vi "ziGetVoltage.vi"(4 "DemodVoltage (Vrms)":cdb[](array[numeric]) format="%#_6p", 6 "ZCtrl / Gain (0)":dbl, 8 "error in":errorcluster, 9 "Demodulator (0)":i32, 10 "Mode":enum16{"From Sig Out", "Signal Input", "HF2CA"}(ring), 11 "handle in":T1 {"Handle" format="0x%08x"; "Conn" format="0x%08x"}) -> (0 "error out":errorcluster, 2 "Vz (Vrms)":cdb[](array[numeric]) format="%#_6p", 3 "handle out":T1 {"Handle" format="0x%08x"; "Conn" format="0x%08x"})   [LabVIEW 2009, in "Zurich Instruments LabOne.lvlib"]
doc: "Get the effective voltage from measured demod samples."
uses:
  <instrlib>/Zurich Instruments LabOne/Zurich Instruments LabOne.lvlib
  <instrlib>/Zurich Instruments LabOne/Public/ziTypeHandle.ctl
  <instrlib>/Zurich Instruments LabOne/Public/Utility/Impedance/ziGetVoltageCalcVec.vi
panel:
  in  "Extra Gain (1)":dbl=1.0
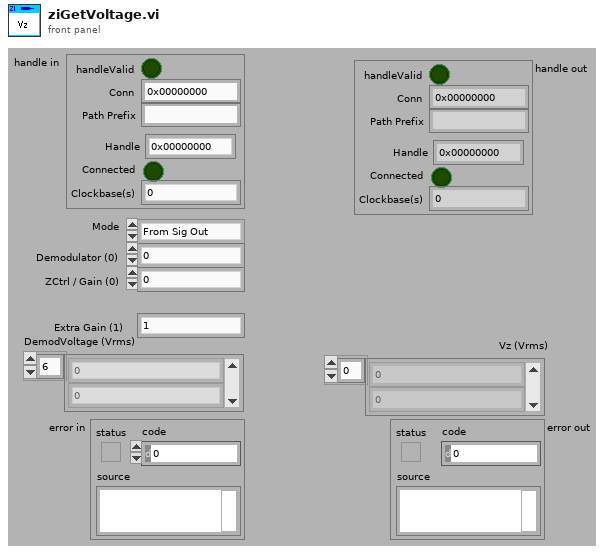
[diagram p1: front panel]
types:
  T1 = typedef "Zurich Instruments LabOne.lvlib/ziTypeHandle.ctl" = cluster{"handleValid":bool, "Conn":u64, "Path Prefix":string, "Handle":u64, "Connected":bool, "Clockbase(s)":dbl}
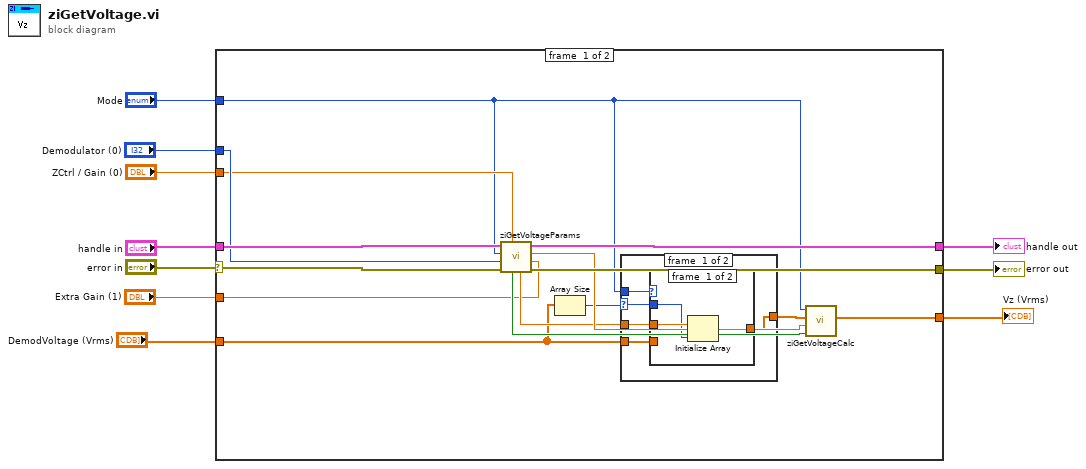
[diagram p0: block diagram]
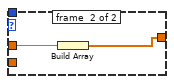
[diagram p3: hidden frame]
diagram:
  n1 = case shown="No Error" "error in" {
    selector: "error in" -> [w23 w37]
    tunnel: "Mode" -> [w11 _]
    tunnel: "ZCtrl / Gain (0)" -> [w17 _]
    tunnel: "handle in" -> [w19 w38]
    tunnel: [w22 _] -> w3
    tunnel: [w25 w38] -> w7
    tunnel: "Demodulator (0)" -> [w18 _]
    tunnel: [w24 w37] -> w5
    tunnel: "DemodVoltage (Vrms)" -> [w14 _]
    tunnel: "Extra Gain (1)" -> [w12 _]
    frame #0 {
      n2 = call <instrlib>:"ziGetVoltageParams.vi"("Extra Gain"=w12, "ZCtrl (0)"=w17, "Error In"=w23, "Demodulator (0)"=w18, "Mode"=w11, "Handle In"=w19) -> ("Error Out"=w24:errorcluster, "VGain"=w21:dbl, "Handle Out"=w25:T1, "Vz (Vrms)"=w16:cdb, "Imp50"=w15:bool)  [unwired: 1 in]
      n3 = Array Size(array=w14) -> (size(s)=w13:i32)
      n4 = case shown="0" w13 {
        selector: w13 -> [w29 _]
        tunnel: [w26 w35] -> w20
        tunnel: w14 -> [w27 _]
        tunnel: w16 -> [w28 w36]
        tunnel: w11 -> [w30 _]
        frame #0 {
          n5 = case shown="Default" w30 {
            tunnel: w29 -> [w32 _]
            tunnel: w28 -> [w33 _]
            tunnel: w27 -> [_ w34]
            tunnel: [w31 w34] -> w26
            frame #0 {
              n6 = Initialize Array(w33, w32) -> (w31:cdb[])
            }
            frame #1 {
            }
          }
        }
        frame #1 {
          n7 = Build Array(w36) -> (w35:cdb[])
        }
      }
      n8 = call-poly <instrlib>:"ziGetVoltageCalc.vi"("Imp50 (F)"=w15, "VGain"=w21, "DemodVoltage (Vrms)"=w20, "Mode"=w11) -> ("Vz (Vrms)"=w22:cdb[])  [unwired: 7 in]
    }
    frame #1 {
    }
  }
  "handle out" <- w7
  "error out" <- w5
  "Vz (Vrms)" <- w3
